vi "Set Up Camera.vi"(11 "error constant":errorcluster) -> ()   [LabVIEW 2014]
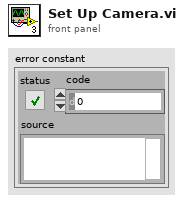
[diagram p1: front panel]
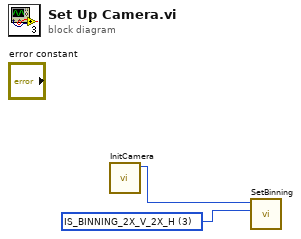
[diagram p0: block diagram]
diagram:
  w1 = 3 items=["IS_BINNING_DISABLE"=0, "IS_BINNING_2X_V"=1, "IS_BINNING_2X_H"=2, "IS_BINNING_4X_V"=4, "IS_BINNING_4X_H"=8, "IS_BINNING_2X_V_2X_H"=3, "IS_BINNING_2X_V_4X_H"=9, "IS_BINNING_4X_V_2X_H"=6, "IS_BINNING_4X_V_4X_H"=12, "IS_GET_BINNING"=32768, "IS_GET_SUPPORTED_BINNING"=32769] ("Mode")
  n1 = call <instrlib>:"InitCamera.vi"() -> ("Camera Handle Out"=w2:u32)  [unwired: 10 in, 1 out]
  n2 = call <instrlib>:"SetBinning.vi"("Mode"=w1, "Camera Handle In"=w2) -> ()  [unwired: 7 in, 3 out]
